vi "Generate graph colours.vi"() -> (2 "Colours":u32[](array[colorbox])=[16777226, 16728642, 982784, 4375295, 13827953, 13457919, 16757522, 4343295, 16728758, 5898228])   [LabVIEW 2017]
panel:
  in  "y":i32(knob)=37854 scale=0.0..50000.0
  out "Add":i32
  out "element":i32
  out "Original index":i32
  out "Color Box":u32(colorbox)
  out "floor(x/y)":i32
  in  "Color Array":u32[](array[colorbox])=[5894143, 15995647, 1703680, 23039, 16121736, 14524158, 16757522, 13628415, 16711686, 2388736, 8956415, 16771626, 16737792, 11796653, 11796497, 10184, 9760512, 9221039, 16755872, 6322771, 16777215, 5374089, 46228, 428288, 1245142, 16751729, 6060418, 8978523, 8879266, 16711680, 13282304]
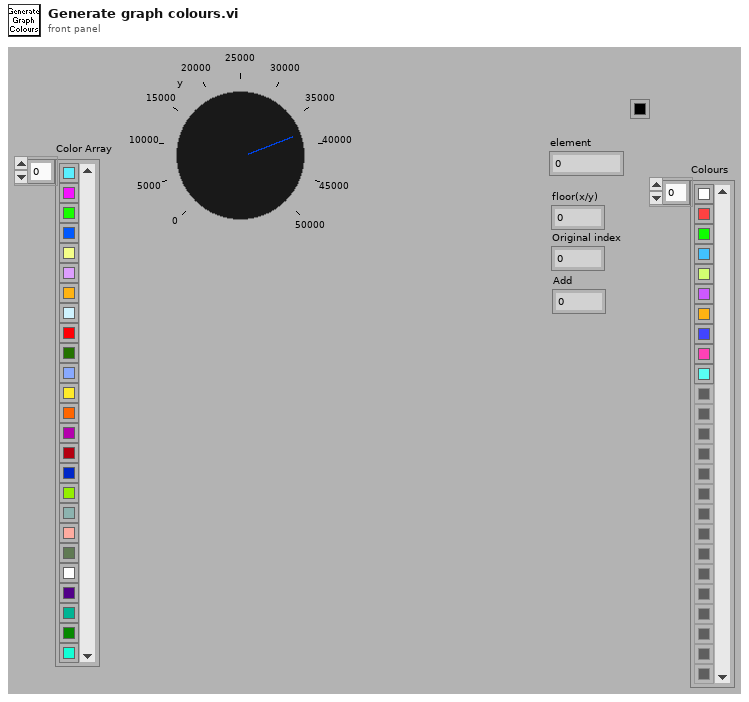
[diagram p1: front panel]
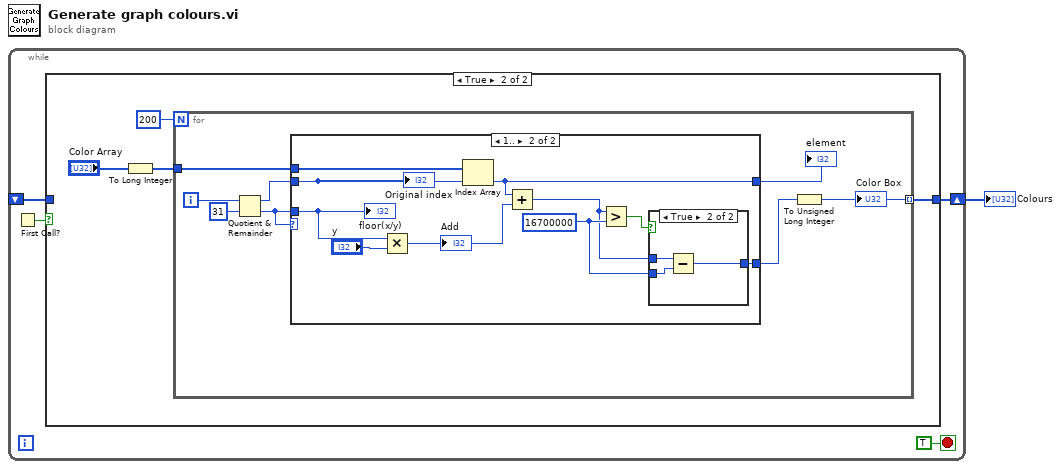
[diagram p0: block diagram]
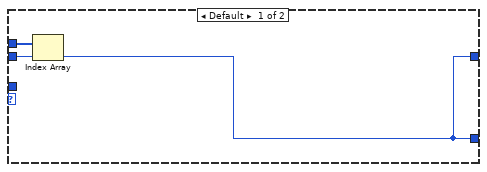
[diagram p3: hidden frame]
diagram:
  n1 = while {
    shift-right: [w5] -> w1
    shift-left: _ -> [w3]
    stop <- TRUE stop-if-true
    n2 = First Call?() -> (First Call?: T/F=w4:bool)
    n3 = case shown="True" w4 {
      tunnel: [w6 w8] -> w5
      tunnel: w3 -> [w6 _]
      frame False {
      }
      frame True {
        n4 = To Long Integer(number="Color Array") -> (32bit integer=w7:i32[])
        n5 = for {
          N: 200 ("Number of plots\nto change color") -> [_]
          tunnel: w7 -> [w17]
          tunnel: [w11] -> w8 mode=indexing
          i -> [w15]
          n6 = Quotient & Remainder(x=w15, y=31) -> (x-y*floor(x/y)=w14:i32, floor(x/y)=w12:i32)
          n7 = case shown="1.." w12 {
            tunnel: w17 -> [w21 w31]
            tunnel: w12 -> [_ w30]
            tunnel: [w19 w29] -> w16
            tunnel: w14 -> [w20 w28]
            tunnel: [w19 w22] -> w13
            frame Default {
              n8 = Index Array(array=w21, index=w20) -> (element=w19:i32)
            }
            frame 1.. {
              w24 = 16700000 ("Numeric")
              n9 = Multiply(x=w30, y="y") -> (x*y=w26:i32)
              "Add" <- w26
              n10 = Index Array(array=w31, index=w28) -> (element=w29:i32)
              n11 = Add(x=w29, y=w26) -> (x+y=w23:i32)
              n12 = Greater?(x=w23, y=w24) -> (0:w25:bool)
              n13 = case shown="True" w25 {
                tunnel: w23 -> [w32 w35]
                tunnel: w24 -> [_ w34]
                tunnel: [w32 w33] -> w22
                frame False {
                }
                frame True {
                  n14 = Subtract(x=w35, y=w34) -> (x-y=w33:i32)
                }
              }
              "floor(x/y)" <- w30
              "Original index" <- w28
            }
          }
          "element" <- w16
          n15 = To Unsigned Long Integer(number=w13) -> (unsigned 32bit integer=w11:u32)
          "Color Box" <- w11
        }
      }
    }
  }
  "Colours" <- w1
